vi "6afft.vi"() -> ()   [LabVIEW 2013]
uses:
  <vilib>/Analysis/2dsp.llb/Real FFT.vi
  <vilib>/Analysis/NI_AALPro.lvlib
panel:
  out "XY Graph":cluster{i32[], "FFT {X}":dbl[]}(graph)
  out "FFT {X}":cdb[](array[numeric])
  in  "Array":string[](array[string])
  # "G SURESH\n23A91A0417\nECE-A"
  # "6A) 8 POINT DISCRETE FOURIER TRANSFROM (DFT)"
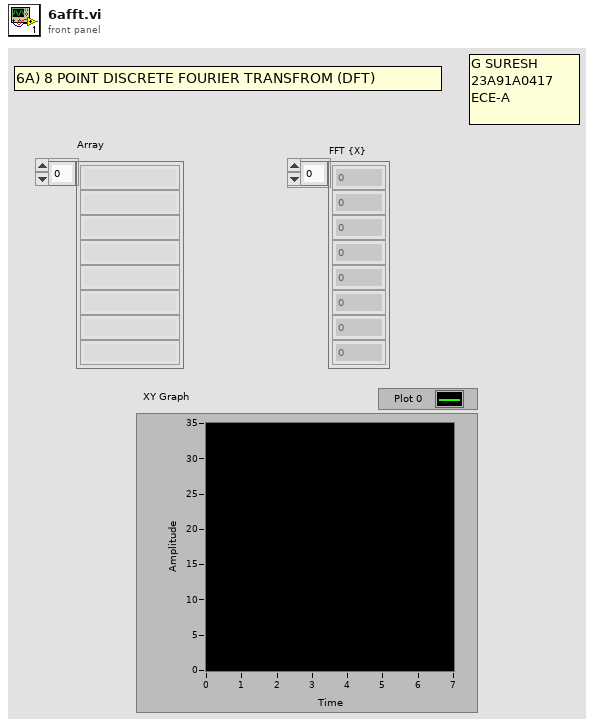
[diagram p1: front panel]
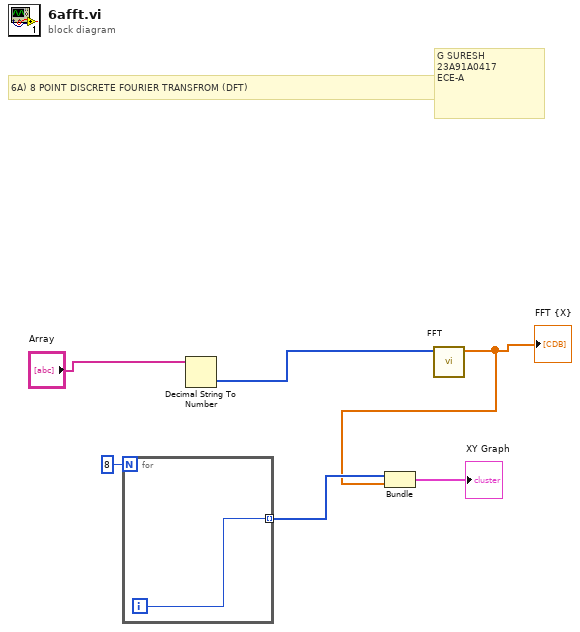
[diagram p0: block diagram]
diagram:
  # "6A) 8 POINT DISCRETE FOURIER TRANSFROM (DFT)"
  # "G SURESH\n23A91A0417\nECE-A"
  n1 = for {
    N: 8 -> [_]
    tunnel: [w7] -> w3 mode=indexing
    i -> [w7]
  }
  n2 = Decimal String To Number(string="Array") -> (number=w5:i32[])  [unwired: 2 in, 1 out]
  n3 = call-poly <vilib>:"FFT.vi"("X"=w5) -> ("FFT {X}"=w2:cdb[])  [unwired: 9 in, 1 out]
  "FFT {X}" <- w2
  n4 = Bundle "Bundle"(w3, "FFT {X}"=w2) -> (→"XY Graph":cluster{i32[], "FFT {X}":cdb[]})  [unwired: 1 in]
